vi "Get Process List.vi"(6 "Invisible Libraries":string[](array[string]), 8 "Error In":errorcluster, 9 "Remove \"System\" library":bool, 11 "Server Name":string="localhost") -> (0 "Error Out":errorcluster, 2 "Libraries":T1, 3 "All Variables":T2)   [LabVIEW 2014]
doc: "<B>Copyright</B>: (c) MHWirth 2015. All rights are reserved.\n\nThis subVI gets the deployed process names and URLs. It can remove those that are specified in \"Invisible Libraries\" from the libraries. Notince the removal is <B>undeployment</B>.\n\nIt also provides all variables info (names + URLs)."
uses:
  <resource>/objmgr/ni.var.rc
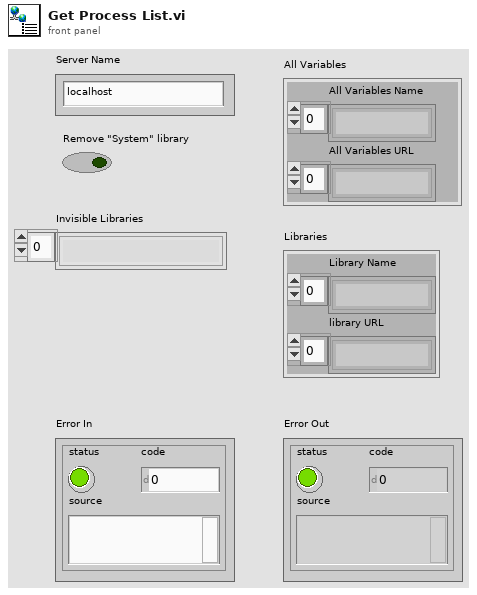
[diagram p1: front panel]
types:
  T1 = cluster{"Library Name":string[], "library URL":string[]}
  T2 = cluster{"All Variables Name":string[], "All Variables URL":string[]}
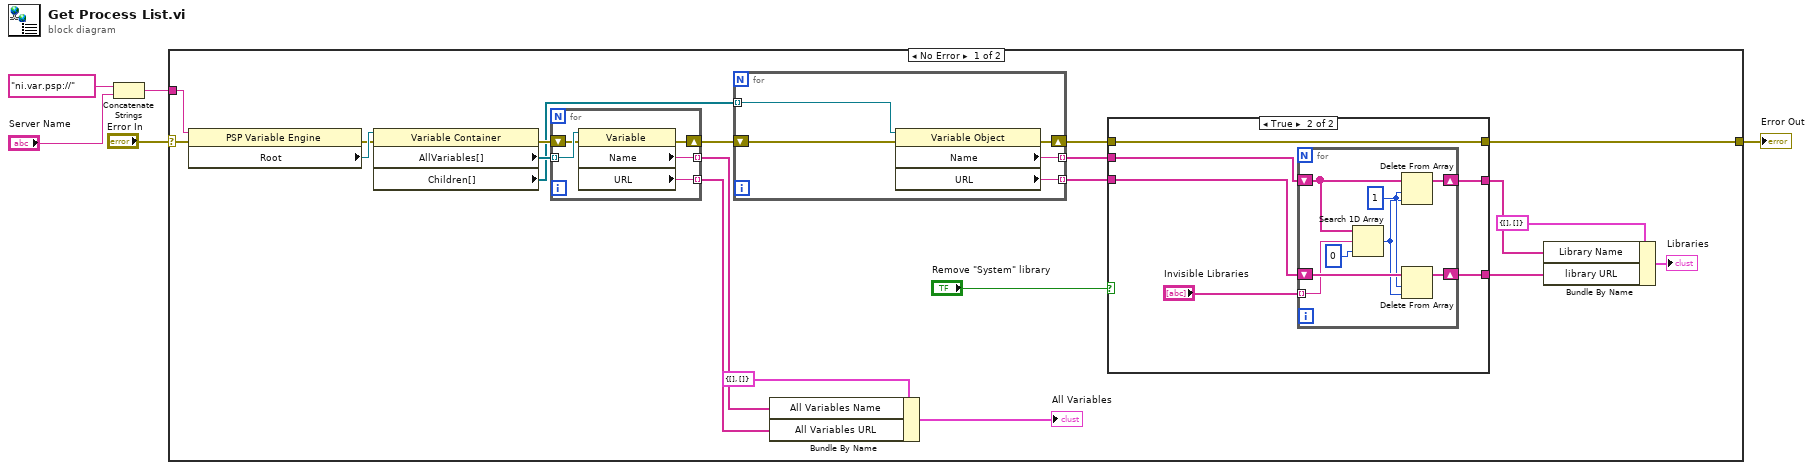
[diagram p0: block diagram]
diagram:
  n1 = Concatenate Strings("ni.var.psp://", "Server Name") -> (w2:string)
  n2 = case shown="No Error" "Error In" {
    selector: "Error In" -> [w24 w54]
    tunnel: w2 -> [w23 _]
    tunnel: [w7 w54] -> w1
    frame No Error {
      n3 = property class="PSP Variable Engine"(reference=w23, error in=w24) -> (error out=w25:errorcluster, "Root"=w26:refnum<k21>)  [unwired: 1 out]
      n4 = property class="Variable Container"(reference=w26, error in=w25) -> (error out=w21:errorcluster, "AllVariables[]"=w22:refnum<k21>[], "Children[]"=w16:refnum<k21>[])  [unwired: 1 out]
      n5 = for {
        tunnel: w22 -> [w53] mode=indexing
        tunnel: [w52] -> w19 mode=indexing
        tunnel: [w51] -> w18 mode=indexing
        shift-right: [w49] -> w17
        shift-left: w21 -> [w50]
        n6 = property class="Variable"(reference=w53, error in=w50) -> (error out=w49:errorcluster, "Name"=w52:string, "URL"=w51:string)  [unwired: 1 out]
      }
      n7 = for {
        tunnel: w16 -> [w48] mode=indexing
        tunnel: [w47] -> w11 mode=indexing
        tunnel: [w46] -> w10 mode=indexing
        shift-right: [w44] -> w6
        shift-left: w17 -> [w45]
        n8 = property class="Variable Object"(reference=w48, error in=w45) -> (error out=w44:errorcluster, "Name"=w47:string, "URL"=w46:string)  [unwired: 1 out]
      }
      n9 = Bundle By Name(cluster=T2 {"All Variables Name"=[], "All Variables URL"=[]}, "All Variables Name"=w19, "All Variables URL"=w18) -> (→"All Variables":T2)
      n10 = case shown="True" "Remove \"System\" library" {
        tunnel: w11 -> [w29 w35]
        tunnel: w10 -> [w28 w34]
        tunnel: [w29 w33] -> w9
        tunnel: [w28 w32] -> w8
        tunnel: [w27 w31] -> w7
        tunnel: w6 -> [w27 w31]
        frame False {
        }
        frame True {
          n11 = for {
            shift-right: [w38] -> w33
            shift-left: w35 -> [w42]
            shift-right: [w37] -> w32
            shift-left: w34 -> [w41]
            tunnel: "Invisible Libraries" -> [w36] mode=indexing
            w40 = 1 ("length")
            n12 = Search 1D Array(1D array=w42, element=w36, start index (0)=0) -> (index of element=w39:i32)
            n13 = Delete From Array(array=w42, length=w40, index=w39) -> (array with subset deleted=w38:string[])  [unwired: 1 out]
            n14 = Delete From Array(array=w41, length=w40, index=w39) -> (array with subset deleted=w37:string[])  [unwired: 1 out]
          }
        }
      }
      n15 = Bundle By Name(cluster=T1 {"Library Name"=[], "library URL"=[]}, "Library Name"=w9, "library URL"=w8) -> (→"Libraries":T1)
    }
    frame Error {
    }
  }
  "Error Out" <- w1
